vi "configuration UI.vi"() -> ()   [LabVIEW 2013, in "EIP Tags editor node.lvclass"]
uses:
  EIP Tags editor node.lvclass
  <vilib>/CEF_TreeControl/Node/NodeRef.ctl
  <vilib>/CEF_TreeControl/Node/NISE_CEF_Node.lvclass
  <vilib>/NI/AMC/Message Queue.ctl
  <vilib>/NI/AMC/Message.ctl
  <vilib>/NI/Tools/Keyed Array/KeyedArray.ctl
  <vilib>/CEF_TreeControl/Node/UserEventRef.ctl
  <vilib>/CEF_TreeControl/Controls/EventCluster.ctl
  <vilib>/NI/Tag Bus Data Framework/Configuration Editor/Classes/Engine Parent/Engine Parent Editor Node.lvclass
  <vilib>/NI/Tag Bus/tag/tag descriptor.lvclass
  <vilib>/NI/Tag Bus/tag/Data Type.ctl
  <vilib>/NI/Module Execution Interface/Engine Configuration/engine configuration.lvclass
  <vilib>/NI/TBM Modules/EIP Tags/configuration/EIP Tags Configuration.lvclass
  <vilib>/NI/Tag Bus/tag/tag descriptor.lvclass/tag descriptor.ctl
  EIP Tags editor node.lvclass/EIP Tags editor node.ctl
  <vilib>/NI/TBM Modules/EIP Tags/configuration/eip tag definition.ctl
  <vilib>/NI/TBM Modules/EIP Tags/configuration/eip tag types.ctl
  <vilib>/NI/Tag Bus Module Framework/root configuration/TBM configuration.lvclass/TBM configuration.ctl
  <vilib>/NI/Tag Bus/tag/write tag name.vi
  <vilib>/NI/Tag Bus/tag/write data type.vi
  <vilib>/NI/Tag Bus Data Framework/Configuration Editor/Classes/Module editor node/Read Module Configuration.vi
  <vilib>/NI/Tag Bus Module Framework/root configuration/create GUID.vi
  <vilib>/NI/Tag Bus Module Framework/module configuration/TBM module configuration.lvclass
  <vilib>/CEF_TreeControl/NISE_CEF_TreeControl.lvlib
  <vilib>/NI/Tag Bus Data Framework/Configuration Editor/Classes/Module editor node/module editor node.lvclass
  <vilib>/NI/Tag Bus Module Framework/root configuration/TBM configuration.lvclass
  <vilib>/NI/Tools/Keyed Array/Tools_KeyedArray.lvlib
  <vilib>/NI/AMC/AMC.lvlib
panel:
  in  "hidden_add":bool
  in  "Tab Control":enum32{"EIP Tags", "Channels"}(tab)
  in  "configure EIPT":bool
  in  "Remove EIPT":bool
  in  "Add EIPT":bool
  in  "EIP tags":i32(listbox)
  in  "Remove Button":bool
  in  "Add Button":bool
  in  "channel":i32(listbox)
  in  "settings":bool
  in  "user event":T1
  in  "main queue":T2
  in  "node ref":T3
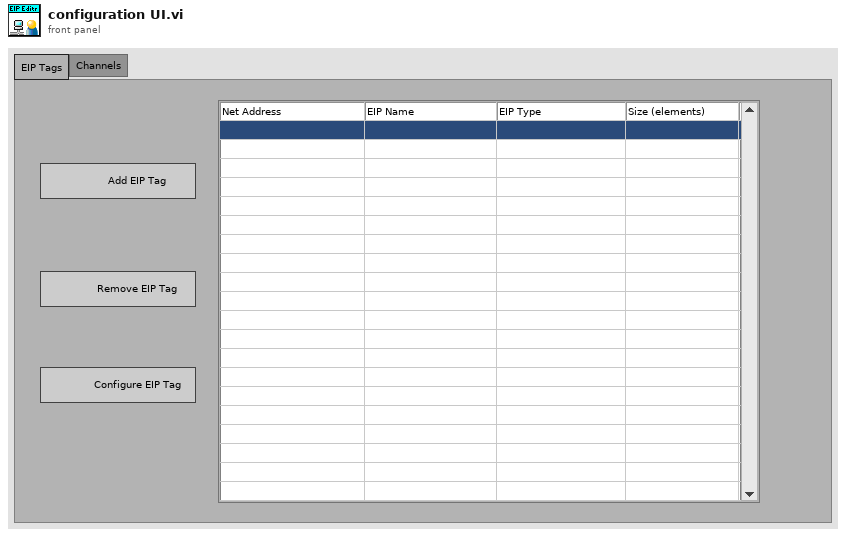
[diagram p1: front panel]
types:
  T1 = typedef "NISE_CEF_Node.lvclass/UserEventRef.ctl" = refnum<user-event>
  T2 = typedef "AMC.lvlib/Message Queue.ctl" = refnum<queue>
  T3 = typedef "NISE_CEF_Node.lvclass/NodeRef.ctl" = refnum<data-value>
  T4 = typedef "NISE_CEF_TreeControl.lvlib/EventCluster.ctl" = cluster{"command":string, "data":string}
  T5 = typedef "tag bus.lvlib/tag descriptor.lvclass/Data Type.ctl" = enum16{"Double", "Single", "I64", "I32", "I16", "I8", "U64", "U32", "U16", "U8", "Boolean", "String", "Array of Double", "Array of Single", "Array of I64", "Array of I32", "Array of I16", "Array of I8", "Array of U64", "Array of U32", "Array of U16", "Array of U8", "Array of Boolean", "Array of String"}
  T6 = typedef "EIP Tags Configuration.lvclass/eip tag definition.ctl" = cluster{"eip tag types":T7, "unique tag name":string, "Number of Elements":u32}
  T7 = typedef "EIP Tags Configuration.lvclass/eip tag types.ctl" = enum16{"SINT", "INT", "DINT", "REAL", "BOOL", "STRING"}
  T8 = typedef "EIP Tags editor node.lvclass/table line.ctl" = cluster{"eip channel":refnum<class "EIP Tags Channel.lvclass">, "tag name":string}
  T9 = typedef "LVPoint32TypeDef.ctl" = cluster{"Horizontal":i32, "Vertical":i32}
  T10 = typedef "LVRowAndColumnTypeDef.ctl" = cluster{"Row":i32, "Column":i32}
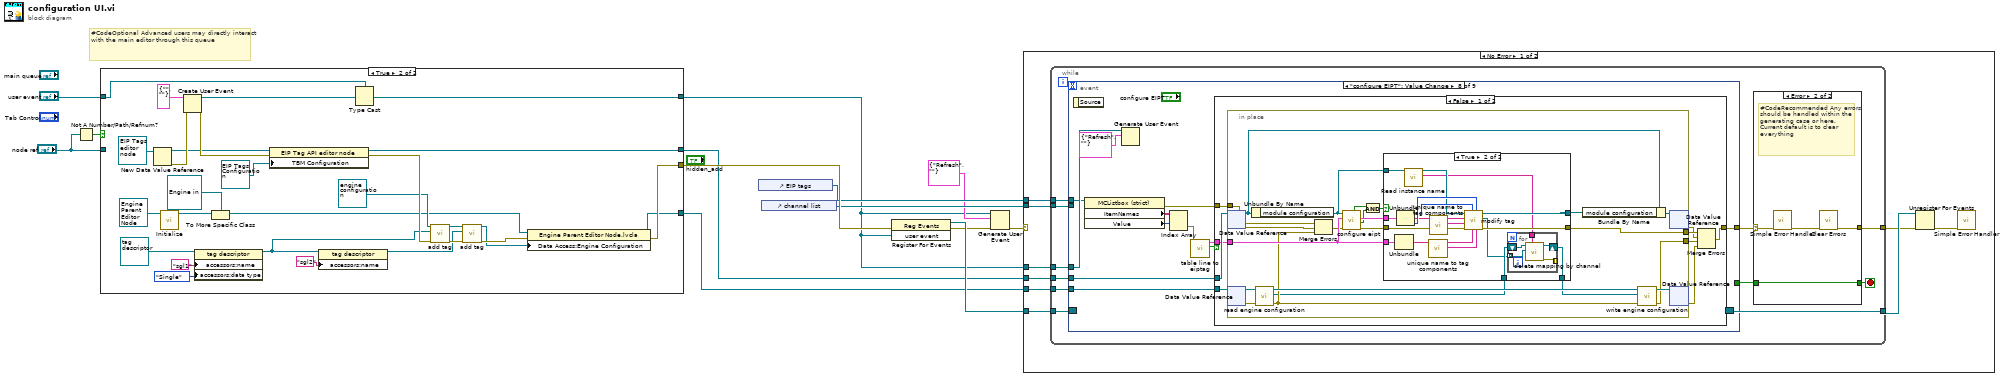
[diagram p0: block diagram]
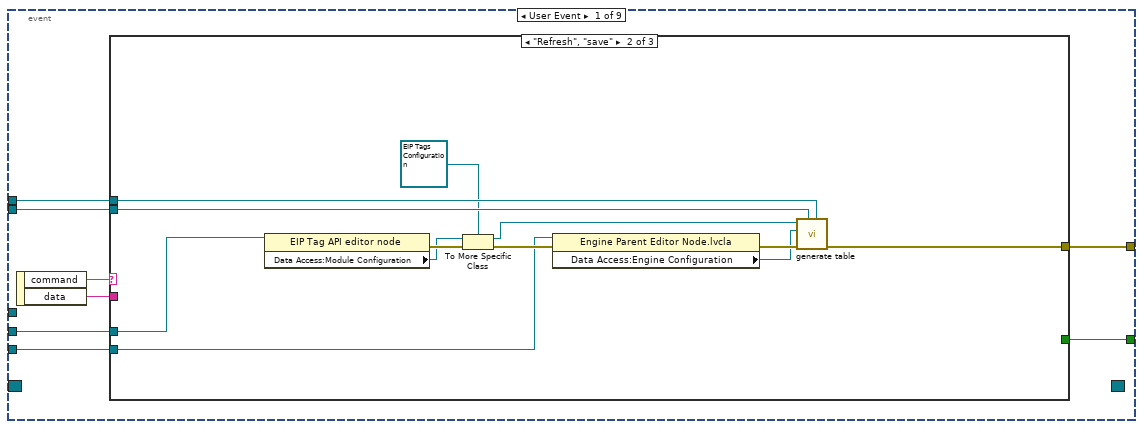
[diagram p3: hidden frame]
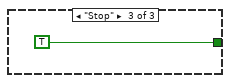
[diagram p5: hidden frame]
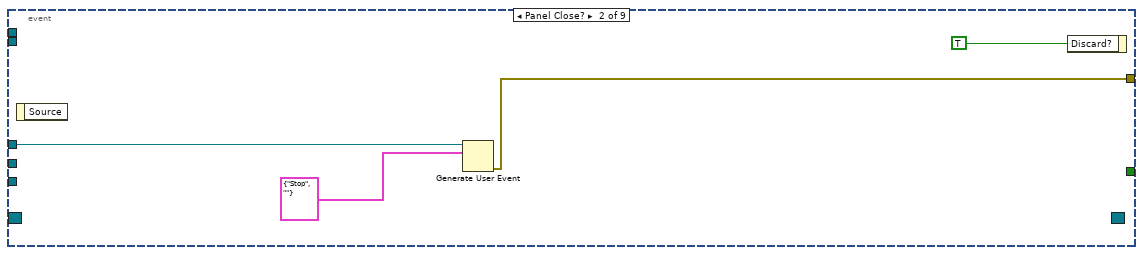
[diagram p6: hidden frame]
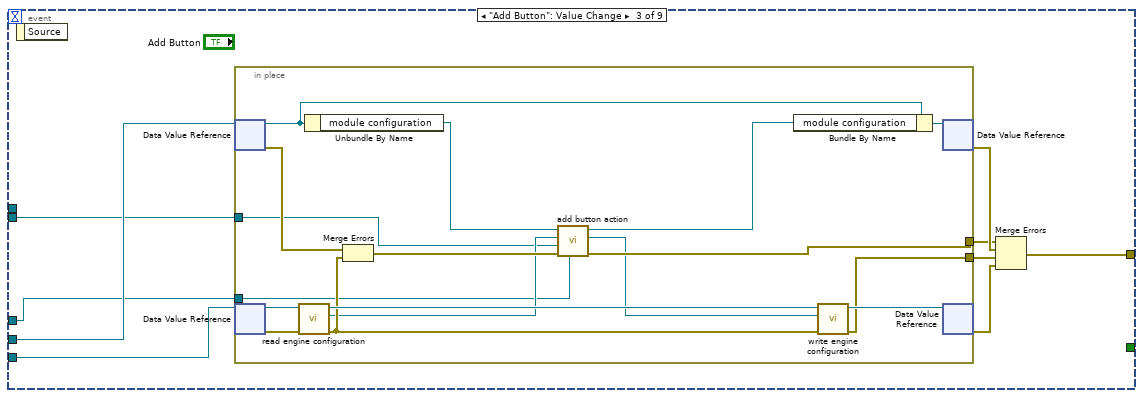
[diagram p7: hidden frame]
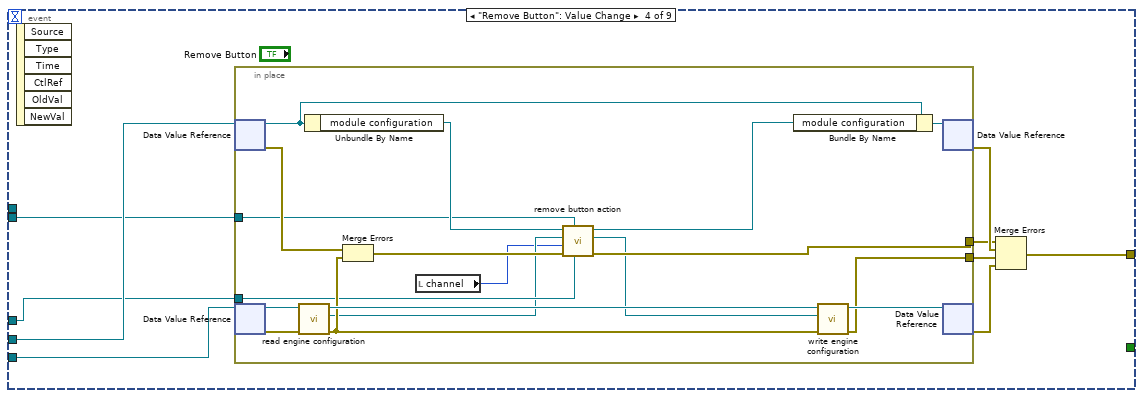
[diagram p8: hidden frame]
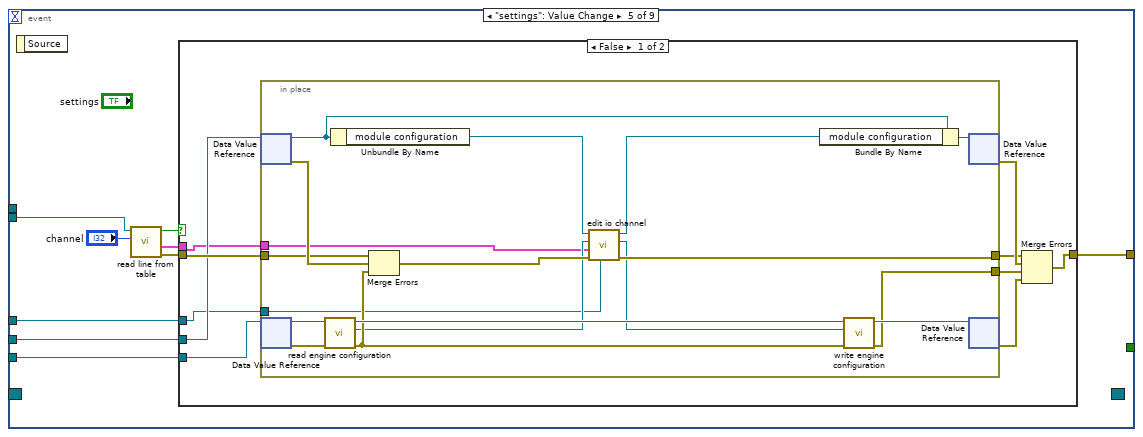
[diagram p9: hidden frame]
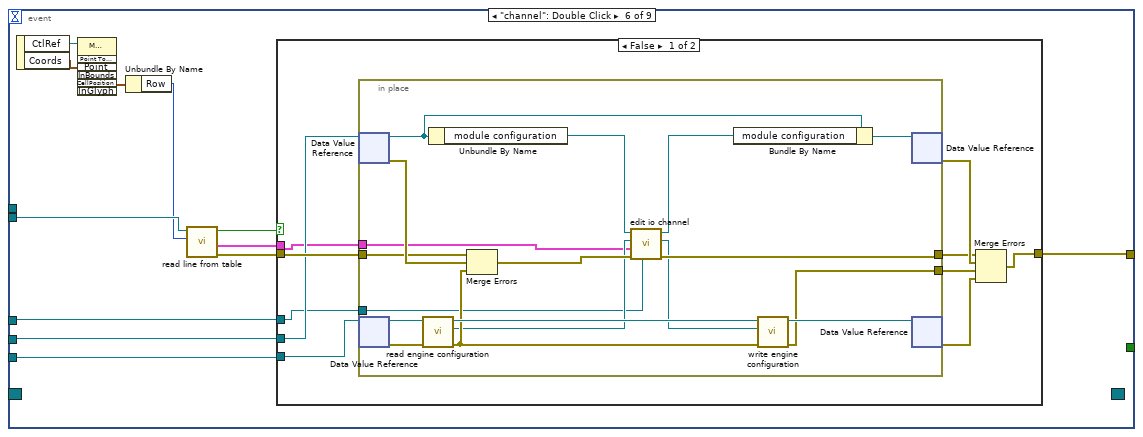
[diagram p11: hidden frame]
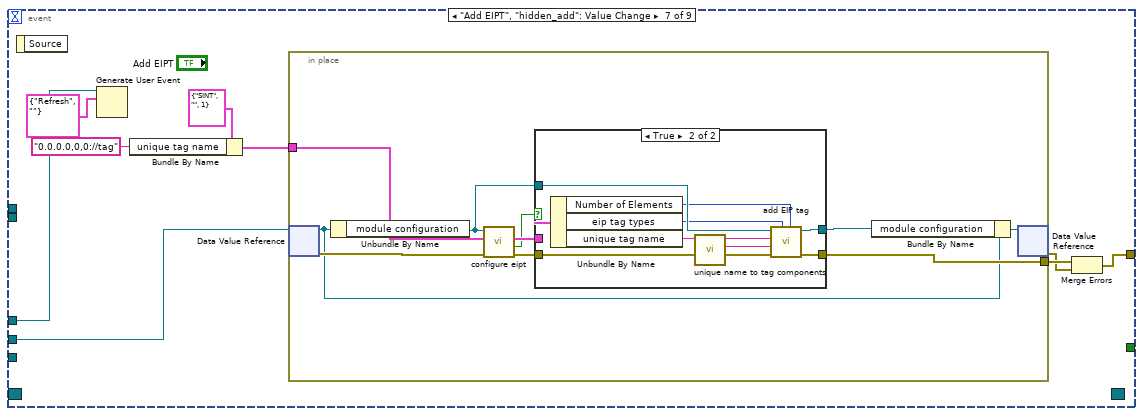
[diagram p13: hidden frame]
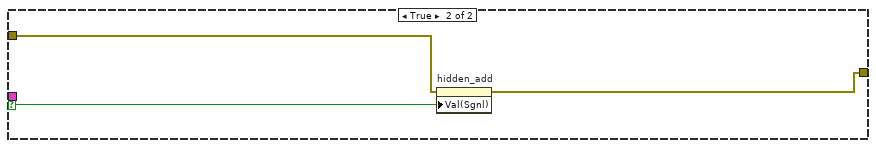
[diagram p16: hidden frame]
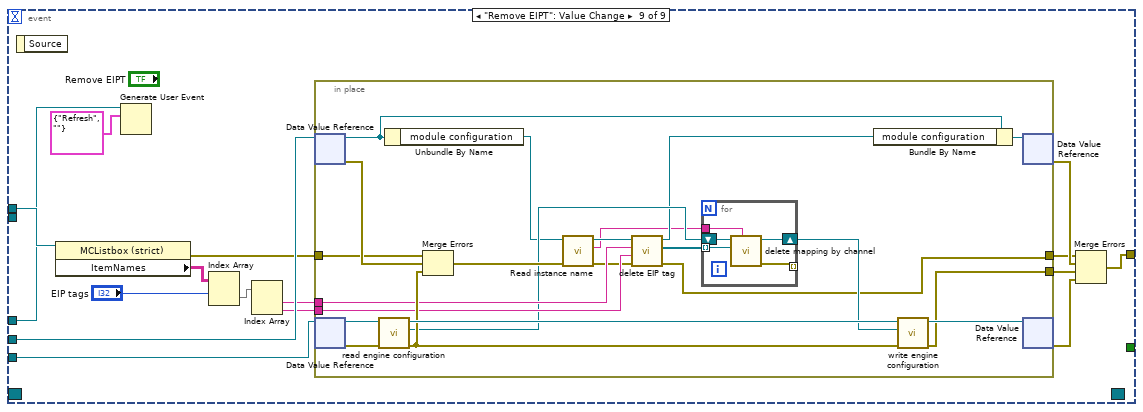
[diagram p17: hidden frame]
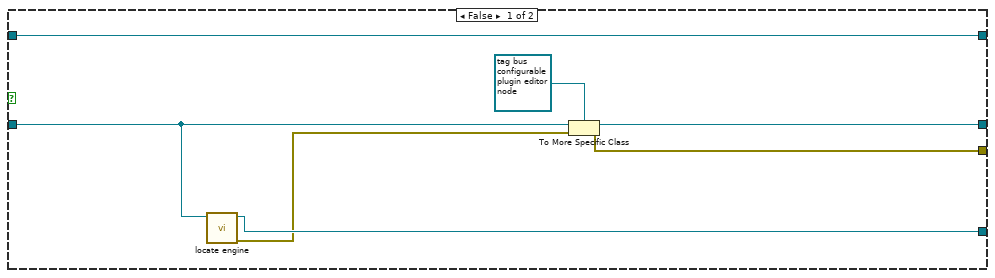
[diagram p19: hidden frame]
diagram:
  # "#CodeOptional Advanced users may directly interact with the main editor through this queue"
  n1 = Not A Number/Path/Refnum?(number/path/refnum="node ref") -> (NaN/Path/Refnum?=w12:bool)
  n2 = case shown="True" w12 {
    tunnel: "user event" -> [w20 w27]
    tunnel: [w20 w28] -> w3
    tunnel: "node ref" -> [w18 _]
    tunnel: [w17 w43] -> w8
    tunnel: [w16 w24] -> w10
    tunnel: [w15 w22] -> w7
    frame False {
      n3 = call <vilib>:"locate engine.vi"("component"=w18) -> ("error out"=w14:errorcluster, "engine"=w15:refnum<data-value>)  [unwired: 9 in]
      n4 = To More Specific Class(target class=refnum<data-value> refnum ("data value reference"), reference=w18, error in=w14) -> (specific class reference=w17:refnum<data-value>, error out=w16:errorcluster)
    }
    frame True {
      n5 = New Data Value Reference(data value=refnum<class "EIP Tags editor node.lvclass"> refnum ("tag bus configurable plugin editor node")) -> (data value reference=w42:refnum<data-value>, error out=w45:errorcluster)  [unwired: 1 in]
      n6 = call-dynamic "Initialize.vi"("Engine in"=refnum<class "Engine Parent Editor Node.lvclass"> refnum) -> ("data value reference"=w41:T3)  [unwired: 8 in, 2 out]
      n7 = Create User Event(user event datatype=T4 {"command"="", "data"=""} ("event data"), error in=w45) -> (user event=w47:refnum<user-event>, error out=w44:errorcluster)
      n8 = property class="tag descriptor"(reference=refnum<class "tag descriptor.lvclass"> refnum ("tag descriptor"), "accessors:name"="sgl1" ("name"), "accessors:data type"=Data_Type."Single" ("data type")) -> (reference out=w29:refnum<class "tag descriptor.lvclass">)  [unwired: 1 in, 1 out]
      n9 = To More Specific Class(target class=refnum<data-value> refnum ("data value reference"), reference=w41) -> (specific class reference=w23:refnum<data-value>)  [unwired: 1 in, 1 out]
      n10 = property class="EIP Tag API editor node"(reference=w42, error in=w44, "TBM Configuration"=refnum<class "EIP Tags Configuration.lvclass"> refnum ("tag bus configurable plugin module configuration")) -> (reference out=w43:refnum<data-value>, error out=w35:errorcluster)
      n11 = property class="tag descriptor"(reference=w29, "accessors:name"="sgl2" ("name")) -> (reference out=w30:refnum<class "tag descriptor.lvclass">)  [unwired: 1 in, 1 out]
      n12 = Type Cast(type=w27, x=w47) -> (*(type *) &x=w28:T1)
      n13 = call <vilib>:"add tag.vi"("error in"=w35, "tag descriptor"=w29, "engine configuration in"=refnum<class "engine configuration.lvclass"> refnum ("Engine Configuration")) -> ("error out"=w33:errorcluster, "engine configuration out"=w32:refnum<class "engine configuration.lvclass">)  [unwired: 7 in]
      n14 = call <vilib>:"add tag.vi"("error in"=w33, "tag descriptor"=w30, "engine configuration in"=w32) -> ("error out"=w31:errorcluster, "engine configuration out"=w21:refnum<class "engine configuration.lvclass">)  [unwired: 7 in]
      n15 = property class="Engine Parent Editor Node.lvcla"(reference=w23, error in=w31, "Data Access:Engine Configuration"=w21) -> (reference out=w22:refnum<data-value>, error out=w24:errorcluster)
    }
  }
  n16 = control-ref of="EIP tags"() -> (w5:refnum<vi>)
  n17 = control-ref of="channel list"() -> (w6:refnum<vi>)
  n18 = register-events(error in=w10, w3) -> (reference out=w13:refnum<event-registration>, error out=w2:errorcluster)  [unwired: 1 in]
  n19 = Generate User Event(user event=w3, event data cluster=T4 {"command"="Refresh", "data"=""} ("event data"), error in=w2) -> (error out=w1:errorcluster)  [unwired: 1 in, 1 out]
  n20 = case shown="No Error" w1 {
    tunnel: w13 -> [w57 _]
    tunnel: w8 -> [w54 _]
    tunnel: w7 -> [w53 _]
    tunnel: w6 -> [w51 _]
    tunnel: w5 -> [w50 _]
    tunnel: w3 -> [w49 _]
    frame No Error {
      n21 = while {
        tunnel: w57 -> [w68]
        tunnel: [w67] -> w56
        tunnel: w54 -> [w63]
        tunnel: w53 -> [w62]
        tunnel: w49 -> [w61]
        tunnel: w51 -> [w59]
        tunnel: w50 -> [w58]
        tunnel: [w64] -> w55
        stop <- w66 stop-if-true
        n22 = event shown="[7] \"configure EIPT\": Value Change" {
          selector: w68 -> [_ _ _ _ _ _ _ _ _]
          dyn-events: [_ _ _ _ _ _ _ _ _] -> w67
          timeout: _ -> [_ _ _ _ _ _ _ _ _]
          tunnel: [w82 _ _ _ _ _ _ _ _] -> w65
          tunnel: [w77 w96 w104 w130 w161 w194 w233 w271 w341] -> w60
          tunnel: w63 -> [w80 _ w102 w128 w153 w192 w234 w272 w339]
          tunnel: w62 -> [w79 _ w103 w129 w154 w191 _ w264 w340]
          tunnel: w61 -> [_ w98 w100 w126 w157 w193 w237 w273 w348]
          tunnel: w59 -> [w76 _ w101 w127 w155 w202 _ _ _]
          tunnel: w58 -> [w75 _ _ _ _ _ _ w270 w351]
          event User Event {
            n23 = event-data() -> ("command"=w81:string, "data"=w78:string)  [unwired: 1 in]
            n24 = case shown="\"Refresh\", \"save\"" w81 {
              tunnel: [_ _ TRUE] -> w82
              tunnel: w80 -> [_ w89 _]
              tunnel: w79 -> [_ w84 _]
              tunnel: w78 -> [_ _ _]
              tunnel: [_ w94 _] -> w77
              tunnel: w76 -> [_ w93 _]
              tunnel: w75 -> [_ w92 _]
              frame Default {
              }
              frame "Refresh", "save" {
                n25 = property class="EIP Tag API editor node"(reference=w89) -> (error out=w90:errorcluster, "Data Access:Module Configuration"=w87:refnum<class "TBM module configuration.lvclass">)  [unwired: 1 in, 1 out]
                n26 = To More Specific Class(target class=refnum<class "EIP Tags Configuration.lvclass"> refnum ("tag bus configurable plugin module configuration"), reference=w87, error in=w90) -> (specific class reference=w85:refnum<class "EIP Tags Configuration.lvclass">, error out=w88:errorcluster)
                n27 = property class="Engine Parent Editor Node.lvcla"(reference=w84, error in=w88) -> (error out=w91:errorcluster, "Data Access:Engine Configuration"=w83:refnum<class "engine configuration.lvclass">)  [unwired: 1 out]
                n28 = call "generate table.vi"("assemblies"=w92, "table"=w93, "error in"=w91, "engine configuration in"=w83, "EthernetIP configuration in"=w85) -> ("error out"=w94:errorcluster)  [unwired: 6 in]
              }
              frame "Stop" {
              }
            }
          }
          event Panel Close? {
            n29 = event-data() -> ()  [unwired: 1 in, 1 out]
            n30 = Generate User Event(user event=w98, event data cluster=T4 {"command"="Stop", "data"=""} ("event data")) -> (error out=w96:errorcluster)  [unwired: 2 in, 1 out]
            n31 = event-data("Discard?"=TRUE) -> ()  [unwired: 1 in, 1 out]
          }
          event "Add Button": Value Change {
            n32 = event-data() -> ()  [unwired: 1 in, 1 out]
            n33 = in-place {
              in-place-border: [w115] -> w105
              in-place-border: [w121] -> w108
              in-place-border: w101 -> [w110]
              in-place-border: w100 -> [w109]
              n34 = in-place-dvr #1(w102) -> (w125:refnum<class "EIP Tags editor node.lvclass">, w123:errorcluster)
              n35 = in-place-dvr #2(w103) -> (w120:refnum<class "Engine Parent Editor Node.lvclass">, w119:errorcluster)
              n36 = call <vilib>:"read engine configuration.vi"("error in"=w119, "Engine Parent Editor Node in"=w120) -> ("error out"=w117:errorcluster, "engine configuration"=w112:refnum<class "engine configuration.lvclass">, "Engine Parent Editor Node out"=w118:refnum<class "Engine Parent Editor Node.lvclass">)  [unwired: 7 in]
              n37 = Unbundle By Name(w125) -> ("module configuration"=w113:refnum<class "EIP Tags Configuration.lvclass">)
              n38 = Merge Errors(w123, w117) -> (w116:errorcluster)
              n39 = call "add button action.vi"("user event"=w109, "error in"=w116, "channel list"=w110, "Engine Configuration"=w112, "EIP Tags Configuration in"=w113) -> ("error out"=w115:errorcluster, "Engine Configuration out"=w111:refnum<class "engine configuration.lvclass">, "module configuration out"=w114:refnum<class "EIP Tags Configuration.lvclass">)  [unwired: 4 in]
              n40 = Bundle By Name(cluster=w125, "module configuration"=w114) -> (w124:refnum<class "EIP Tags editor node.lvclass">)
              n41 = call <vilib>:"write engine configuration.vi"("error in"=w117, "engine configuration"=w111, "Engine Parent Editor Node in"=w118) -> ("error out"=w121:errorcluster, "Engine Parent Editor Node out"=w122:refnum<class "Engine Parent Editor Node.lvclass">)  [unwired: 7 in]
              n42 = in-place-dvr #1(w124) -> (w107:errorcluster)  [unwired: 1 out]
              n43 = in-place-dvr #2(w122) -> (w106:errorcluster)  [unwired: 1 out]
            }
            n44 = Merge Errors(w105, w107, w108, w106) -> (w104:errorcluster)
          }
          event "Remove Button": Value Change {
            n45 = event-data() -> ()  [unwired: 1 in, 6 out]
            n46 = in-place {
              in-place-border: [w142] -> w131
              in-place-border: [w148] -> w134
              in-place-border: w127 -> [w138]
              in-place-border: w126 -> [w141]
              n47 = in-place-dvr #3(w128) -> (w152:refnum<class "EIP Tags editor node.lvclass">, w150:errorcluster)
              n48 = in-place-dvr #4(w129) -> (w147:refnum<class "Engine Parent Editor Node.lvclass">, w146:errorcluster)
              n49 = call <vilib>:"read engine configuration.vi"("error in"=w146, "Engine Parent Editor Node in"=w147) -> ("error out"=w144:errorcluster, "engine configuration"=w137:refnum<class "engine configuration.lvclass">, "Engine Parent Editor Node out"=w145:refnum<class "Engine Parent Editor Node.lvclass">)  [unwired: 7 in]
              n50 = Unbundle By Name(w152) -> ("module configuration"=w139:refnum<class "EIP Tags Configuration.lvclass">)
              n51 = Merge Errors(w150, w144) -> (w143:errorcluster)
              n52 = local read "channel"() -> (w135:i32)
              n53 = call "remove button action.vi"("user event"=w141, "channel list"=w138, "error in"=w143, "channel"=w135, "Engine Configuration in"=w137, "EIP Tags Configuration in"=w139) -> ("error out"=w142:errorcluster, "Engine Configuration out"=w136:refnum<class "engine configuration.lvclass">, "EIP Tags Configuration out"=w140:refnum<class "EIP Tags Configuration.lvclass">)  [unwired: 3 in]
              n54 = Bundle By Name(cluster=w152, "module configuration"=w140) -> (w151:refnum<class "EIP Tags editor node.lvclass">)
              n55 = call <vilib>:"write engine configuration.vi"("error in"=w144, "engine configuration"=w136, "Engine Parent Editor Node in"=w145) -> ("error out"=w148:errorcluster, "Engine Parent Editor Node out"=w149:refnum<class "Engine Parent Editor Node.lvclass">)  [unwired: 7 in]
              n56 = in-place-dvr #3(w151) -> (w133:errorcluster)  [unwired: 1 out]
              n57 = in-place-dvr #4(w149) -> (w132:errorcluster)  [unwired: 1 out]
            }
            n58 = Merge Errors(w131, w133, w134, w132) -> (w130:errorcluster)
          }
          event "settings": Value Change {
            n59 = event-data() -> ()  [unwired: 1 in, 1 out]
            n60 = call "read line from table.vi"("line number"="channel", "channels table"=w155) -> ("error out"=w160:errorcluster, "line"=w159:T8, "empty channel?"=w156:bool)  [unwired: 6 in, 1 out]
            n61 = case shown="False" w156 {
              tunnel: [w167 w190] -> w161
              tunnel: w160 -> [w166 w190]
              tunnel: w159 -> [w163 _]
              tunnel: w157 -> [w162 _]
              tunnel: w154 -> [w165 _]
              tunnel: w153 -> [w164 _]
              frame False {
                n62 = in-place {
                  in-place-border: [w178] -> w168
                  in-place-border: [w185] -> w171
                  in-place-border: w166 -> [w180]
                  in-place-border: w163 -> [w173]
                  in-place-border: w162 -> [w172]
                  n63 = in-place-dvr #5(w164) -> (w189:refnum<class "EIP Tags editor node.lvclass">, w187:errorcluster)
                  n64 = in-place-dvr #6(w165) -> (w184:refnum<class "Engine Parent Editor Node.lvclass">, w183:errorcluster)
                  n65 = call <vilib>:"read engine configuration.vi"("error in"=w183, "Engine Parent Editor Node in"=w184) -> ("error out"=w181:errorcluster, "engine configuration"=w174:refnum<class "engine configuration.lvclass">, "Engine Parent Editor Node out"=w182:refnum<class "Engine Parent Editor Node.lvclass">)  [unwired: 7 in]
                  n66 = Unbundle By Name(w189) -> ("module configuration"=w177:refnum<class "EIP Tags Configuration.lvclass">)
                  n67 = Merge Errors(w180, w187, w181) -> (w179:errorcluster)
                  n68 = call "edit io channel.vi"("user event"=w172, "error in"=w179, "line"=w173, "engine configuration in"=w174, "EthernetIP configuration in"=w177) -> ("error out"=w178:errorcluster, "engine configuration out"=w175:refnum<class "engine configuration.lvclass">, "EthernetIP configuration out"=w176:refnum<class "EIP Tags Configuration.lvclass">)  [unwired: 4 in]
                  n69 = Bundle By Name(cluster=w189, "module configuration"=w176) -> (w188:refnum<class "EIP Tags editor node.lvclass">)
                  n70 = call <vilib>:"write engine configuration.vi"("error in"=w181, "engine configuration"=w175, "Engine Parent Editor Node in"=w182) -> ("error out"=w185:errorcluster, "Engine Parent Editor Node out"=w186:refnum<class "Engine Parent Editor Node.lvclass">)  [unwired: 7 in]
                  n71 = in-place-dvr #5(w188) -> (w170:errorcluster)  [unwired: 1 out]
                  n72 = in-place-dvr #6(w186) -> (w169:errorcluster)  [unwired: 1 out]
                }
                n73 = Merge Errors(w168, w170, w171, w169) -> (w167:errorcluster)
              }
              frame True {
              }
            }
          }
          event "channel": Double Click {
            n74 = event-data() -> ("CtlRef"=w201:refnum<vi>, "Coords"=w200:T9)  [unwired: 1 in]
            n75 = invoke class="MCListbox (strict)" method="Point To Row Column"(reference=w201, "Point"=w200) -> ("CellPosition"=w199:T10)  [unwired: 5 in, 6 out]
            n76 = Unbundle By Name(w199) -> ("Row"=w198:i32)
            n77 = call "read line from table.vi"("line number"=w198, "channels table"=w202) -> ("error out"=w197:errorcluster, "line"=w196:T8, "empty channel?"=w195:bool)  [unwired: 6 in, 1 out]
            n78 = case shown="False" w195 {
              tunnel: [w208 w231] -> w194
              tunnel: w197 -> [w207 w231]
              tunnel: w196 -> [w204 _]
              tunnel: w193 -> [w203 _]
              tunnel: w191 -> [w206 _]
              tunnel: w192 -> [w205 _]
              frame False {
                n79 = in-place {
                  in-place-border: [w219] -> w209
                  in-place-border: [w226] -> w212
                  in-place-border: w207 -> [w221]
                  in-place-border: w204 -> [w214]
                  in-place-border: w203 -> [w213]
                  n80 = in-place-dvr #7(w205) -> (w230:refnum<class "EIP Tags editor node.lvclass">, w228:errorcluster)
                  n81 = in-place-dvr #8(w206) -> (w225:refnum<class "Engine Parent Editor Node.lvclass">, w224:errorcluster)
                  n82 = call <vilib>:"read engine configuration.vi"("error in"=w224, "Engine Parent Editor Node in"=w225) -> ("error out"=w222:errorcluster, "engine configuration"=w215:refnum<class "engine configuration.lvclass">, "Engine Parent Editor Node out"=w223:refnum<class "Engine Parent Editor Node.lvclass">)  [unwired: 7 in]
                  n83 = Unbundle By Name(w230) -> ("module configuration"=w218:refnum<class "EIP Tags Configuration.lvclass">)
                  n84 = Merge Errors(w221, w228, w222) -> (w220:errorcluster)
                  n85 = call "edit io channel.vi"("user event"=w213, "error in"=w220, "line"=w214, "engine configuration in"=w215, "EthernetIP configuration in"=w218) -> ("error out"=w219:errorcluster, "engine configuration out"=w216:refnum<class "engine configuration.lvclass">, "EthernetIP configuration out"=w217:refnum<class "EIP Tags Configuration.lvclass">)  [unwired: 4 in]
                  n86 = Bundle By Name(cluster=w230, "module configuration"=w217) -> (w229:refnum<class "EIP Tags editor node.lvclass">)
                  n87 = call <vilib>:"write engine configuration.vi"("error in"=w222, "engine configuration"=w216, "Engine Parent Editor Node in"=w223) -> ("error out"=w226:errorcluster, "Engine Parent Editor Node out"=w227:refnum<class "Engine Parent Editor Node.lvclass">)  [unwired: 7 in]
                  n88 = in-place-dvr #7(w229) -> (w211:errorcluster)  [unwired: 1 out]
                  n89 = in-place-dvr #8(w227) -> (w210:errorcluster)  [unwired: 1 out]
                }
                n90 = Merge Errors(w209, w211, w212, w210) -> (w208:errorcluster)
              }
              frame True {
              }
            }
          }
          event "Add EIPT", "hidden_add": Value Change {
            n91 = event-data() -> ()  [unwired: 1 in, 1 out]
            n92 = Generate User Event(user event=w237, event data cluster=T4 {"command"="Refresh", "data"=""} ("event data")) -> ()  [unwired: 2 in, 2 out]
            n93 = Bundle By Name(cluster=T6 {"eip tag types"=enum."SINT", "unique tag name"="", "Number of Elements"=1} ("tag spec"), "unique tag name"="0.0.0.0,0,0://tag") -> (w239:T6)
            n94 = in-place {
              in-place-border: [w249] -> w240
              in-place-border: w239 -> [w246]
              n95 = in-place-dvr #9(w234) -> (w243:refnum<class "EIP Tags editor node.lvclass">, w245:errorcluster)
              n96 = Unbundle By Name(w243) -> ("module configuration"=w241:refnum<class "EIP Tags Configuration.lvclass">)
              n97 = call "configure eipt.vi"("error in"=w245, "tag definition in"=w246, "EthernetIP configuration"=w241) -> ("error out"=w250:errorcluster, "success"=w247:bool, "tag definition out"=w248:T6)  [unwired: 5 in, 1 out]
              n98 = case shown="True" w247 {
                tunnel: w250 -> [w251 w262]
                tunnel: [w251 w261] -> w249
                tunnel: [w252 w260] -> w242
                tunnel: w241 -> [w252 w259]
                tunnel: w248 -> [_ w258]
                frame False {
                }
                frame True {
                  n99 = Unbundle By Name(w258) -> ("Number of Elements"=w256:u32, "eip tag types"=w257:T7, "unique tag name"=w255:string)
                  n100 = call <vilib>:"unique name to tag components.vi"("unique name"=w255) -> ("Tag Name"=w253:string, "Network Path"=w254:string)  [unwired: 9 in]
                  n101 = call <vilib>:"add EIP tag.vi"("Number of Elements"=w256, "eip tag types"=w257, "error in"=w262, "Tag Name"=w253, "Network Path"=w254, "EIP Tags configuration in"=w259) -> ("error out"=w261:errorcluster, "EIP Tags configuration out"=w260:refnum<class "EIP Tags Configuration.lvclass">)  [unwired: 4 in]
                }
              }
              n102 = Bundle By Name(cluster=w243, "module configuration"=w242) -> (w244:refnum<class "EIP Tags editor node.lvclass">)
              n103 = in-place-dvr #9(w244) -> (w232:errorcluster)  [unwired: 1 out]
            }
            n104 = Merge Errors(w240, w232) -> (w233:errorcluster)
          }
          event "configure EIPT": Value Change {
            n105 = event-data() -> ()  [unwired: 1 in, 1 out]
            n106 = property class="MCListbox (strict)"(reference=w270) -> (error out=w263:errorcluster, "ItemNames"=w269:string[][], "Value"=w268:i32)  [unwired: 1 in, 1 out]
            n107 = Generate User Event(user event=w273, event data cluster=T4 {"command"="Refresh", "data"=""} ("event data")) -> ()  [unwired: 2 in, 2 out]
            n108 = Index Array(array=w269, index (row)=w268) -> (element=w267:string[])  [unwired: 1 in]
            n109 = call "table line to eiptag.vi"("line strings"=w267) -> ("invalid?"=w266:bool, "tag"=w265:T6)  [unwired: 9 in]
            n110 = case shown="False" w266 {
              selector: w266 -> [_ w335]
              tunnel: w272 -> [w282 _]
              tunnel: [w281 w334] -> w271
              tunnel: w265 -> [w279 _]
              tunnel: w264 -> [w278 _]
              tunnel: w263 -> [w275 w333]
              frame False {
                n111 = in-place {
                  in-place-border: [w304] -> w283
                  in-place-border: w279 -> [w294]
                  in-place-border: [w287] -> w276
                  in-place-border: w275 -> [w284]
                  n112 = in-place-dvr #10(w282) -> (w300:refnum<class "EIP Tags editor node.lvclass">, w302:errorcluster)
                  n113 = in-place-dvr #11(w278) -> (w293:refnum<class "Engine Parent Editor Node.lvclass">, w292:errorcluster)
                  n114 = Unbundle By Name(w300) -> ("module configuration"=w298:refnum<class "EIP Tags Configuration.lvclass">)
                  n115 = call <vilib>:"read engine configuration.vi"("error in"=w292, "Engine Parent Editor Node in"=w293) -> ("error out"=w288:errorcluster, "engine configuration"=w286:refnum<class "engine configuration.lvclass">, "Engine Parent Editor Node out"=w289:refnum<class "Engine Parent Editor Node.lvclass">)  [unwired: 7 in]
                  n116 = Merge Errors(w284, w302, w288) -> (w291:errorcluster)
                  n117 = call "configure eipt.vi"("error in"=w291, "tag definition in"=w294, "EthernetIP configuration"=w298) -> ("error out"=w305:errorcluster, "success"=w295:bool, "tag definition out"=w303:T6, "changed"=w296:bool)  [unwired: 5 in]
                  n118 = And(x=w296, y=w295) -> (x .and. y?=w297:bool)
                  n119 = case shown="True" w297 {
                    tunnel: w305 -> [w307 w327]
                    tunnel: [w307 w326] -> w304
                    tunnel: [w308 w325] -> w299
                    tunnel: w298 -> [w308 w312]
                    tunnel: w303 -> [_ w323]
                    tunnel: w294 -> [_ w324]
                    tunnel: w286 -> [w306 w314]
                    tunnel: [w306 w313] -> w285
                    frame False {
                    }
                    frame True {
                      n120 = Unbundle(w324) -> ("unique tag name"=w317:string)  [unwired: 2 out]
                      n121 = Unbundle(w323) -> ("eip tag types"=w321:T7, "unique tag name"=w320:string, "Number of Elements"=w322:u32)
                      n122 = call <vilib>:"Read instance name.vi"("configuration in"=w312) -> ("instance id"=w310:string, "configuration out"=w311:refnum<class "EIP Tags Configuration.lvclass">)  [unwired: 8 in, 1 out]
                      n123 = call <vilib>:"unique name to tag components.vi"("unique name"=w317) -> ("Tag Name"=w315:string, "Network Path"=w316:string)  [unwired: 9 in]
                      n124 = call <vilib>:"unique name to tag components.vi"("unique name"=w320) -> ("Tag Name"=w318:string, "Network Path"=w319:string)  [unwired: 9 in]
                      n125 = call <vilib>:"modify tag.vi"("original tag name"=w315, "Number of Elements"=w322, "original network path"=w316, "eip tag types"=w321, "error in"=w327, "Tag Name"=w318, "Network Path"=w319, "EIP Tags configuration in"=w311) -> ("error out"=w326:errorcluster, "removed channels"=w309:refnum<class "EIP Tags Channel.lvclass">[], "EIP Tags configuration out"=w325:refnum<class "EIP Tags Configuration.lvclass">)  [unwired: 1 in]
                      n126 = for {
                        shift-right: [w332] -> w313
                        shift-left: w314 -> [w331]
                        tunnel: [w330] -> _ mode=indexing
                        tunnel: w310 -> [w329]
                        tunnel: w309 -> [w328] mode=indexing
                        n127 = call <vilib>:"delete mapping by channel.vi"("owner ID"=w329, "channel"=w328, "engine configuration in"=w331) -> ("error out"=w330:errorcluster, "engine configuration out"=w332:refnum<class "engine configuration.lvclass">)  [unwired: 7 in]
                      }
                    }
                  }
                  n128 = Bundle By Name(cluster=w300, "module configuration"=w299) -> (w301:refnum<class "EIP Tags editor node.lvclass">)
                  n129 = call <vilib>:"write engine configuration.vi"("error in"=w288, "engine configuration"=w285, "Engine Parent Editor Node in"=w289) -> ("error out"=w287:errorcluster, "Engine Parent Editor Node out"=w290:refnum<class "Engine Parent Editor Node.lvclass">)  [unwired: 7 in]
                  n130 = in-place-dvr #10(w301) -> (w280:errorcluster)  [unwired: 1 out]
                  n131 = in-place-dvr #11(w290) -> (w277:errorcluster)  [unwired: 1 out]
                }
                n132 = Merge Errors(w283, w280, w276, w277) -> (w281:errorcluster)
              }
              frame True {
                n133 = property on="hidden_add" class="Bool (strict)"(error in=w333, "Val(Sgnl)"=w335) -> (error out=w334:errorcluster)  [unwired: 1 in, 1 out]
              }
            }
          }
          event "Remove EIPT": Value Change {
            n134 = event-data() -> ()  [unwired: 1 in, 1 out]
            n135 = property class="MCListbox (strict)"(reference=w351) -> (error out=w338:errorcluster, "ItemNames"=w350:string[][])  [unwired: 1 in, 1 out]
            n136 = Generate User Event(user event=w348, event data cluster=T4 {"command"="Refresh", "data"=""} ("event data")) -> ()  [unwired: 2 in, 2 out]
            n137 = Index Array(array=w350, index (row)="EIP tags") -> (element=w346:string[])  [unwired: 1 in]
            n138 = Index Array(array=w346) -> (element #1=w337:string, element #2=w336:string)  [unwired: 2 in]
            n139 = in-place {
              in-place-border: [w352] -> w342
              in-place-border: [w369] -> w345
              in-place-border: w338 -> [w364]
              in-place-border: w337 -> [w362]
              in-place-border: w336 -> [w361]
              n140 = in-place-dvr #12(w339) -> (w373:refnum<class "EIP Tags editor node.lvclass">, w371:errorcluster)
              n141 = in-place-dvr #13(w340) -> (w368:refnum<class "Engine Parent Editor Node.lvclass">, w367:errorcluster)
              n142 = call <vilib>:"read engine configuration.vi"("error in"=w367, "Engine Parent Editor Node in"=w368) -> ("error out"=w365:errorcluster, "engine configuration"=w360:refnum<class "engine configuration.lvclass">, "Engine Parent Editor Node out"=w366:refnum<class "Engine Parent Editor Node.lvclass">)  [unwired: 7 in]
              n143 = Unbundle By Name(w373) -> ("module configuration"=w357:refnum<class "EIP Tags Configuration.lvclass">)
              n144 = Merge Errors(w364, w371, w365) -> (w363:errorcluster)
              n145 = call <vilib>:"Read instance name.vi"("error in"=w363, "configuration in"=w357) -> ("error out"=w355:errorcluster, "instance id"=w353:string, "configuration out"=w354:refnum<class "EIP Tags Configuration.lvclass">)  [unwired: 7 in]
              n146 = call <vilib>:"delete EIP tag.vi"("error in"=w355, "Tag Name"=w361, "Network Path"=w362, "EIP Tags configuration in"=w354) -> ("error out"=w352:errorcluster, "removed channels"=w356:refnum<class "EIP Tags Channel.lvclass">[], "EIP Tags configuration out"=w358:refnum<class "EIP Tags Configuration.lvclass">)  [unwired: 5 in]
              n147 = for {
                shift-right: [w378] -> w359
                shift-left: w360 -> [w377]
                tunnel: w356 -> [w376] mode=indexing
                tunnel: [w375] -> _ mode=indexing
                tunnel: w353 -> [w374]
                n148 = call <vilib>:"delete mapping by channel.vi"("owner ID"=w374, "channel"=w376, "engine configuration in"=w377) -> ("error out"=w375:errorcluster, "engine configuration out"=w378:refnum<class "engine configuration.lvclass">)  [unwired: 7 in]
              }
              n149 = Bundle By Name(cluster=w373, "module configuration"=w358) -> (w372:refnum<class "EIP Tags editor node.lvclass">)
              n150 = call <vilib>:"write engine configuration.vi"("error in"=w365, "engine configuration"=w359, "Engine Parent Editor Node in"=w366) -> ("error out"=w369:errorcluster, "Engine Parent Editor Node out"=w370:refnum<class "Engine Parent Editor Node.lvclass">)  [unwired: 7 in]
              n151 = in-place-dvr #12(w372) -> (w344:errorcluster)  [unwired: 1 out]
              n152 = in-place-dvr #13(w370) -> (w343:errorcluster)  [unwired: 1 out]
            }
            n153 = Merge Errors(w342, w344, w345, w343) -> (w341:errorcluster)
          }
        }
        n154 = case shown="Error" w60 {
          selector: w60 -> [w69 w73]
          tunnel: [w70 w74] -> w66
          tunnel: w65 -> [w70 w74]
          tunnel: [w69 w71] -> w64
          frame No Error {
          }
          frame Error {
            # "#CodeRecommended Any errors should be handled within the generating case or here. Current default is to clear everything"
            n155 = call <vilib>:"Simple Error Handler.vi"("error in (no error)"=w73) -> ("error out"=w72:errorcluster)  [unwired: 4 in, 4 out]
            n156 = call <vilib>:"Clear Errors.vi"("error in (no error)"=w72) -> ("error out"=w71:errorcluster)  [unwired: 6 in]
          }
        }
      }
      n157 = Unregister For Events(event registration refnum=w56, error in=w55) -> (error out=w52:errorcluster)
      n158 = call <vilib>:"Simple Error Handler.vi"("error in (no error)"=w52) -> ()  [unwired: 4 in, 5 out]
    }
    frame Error {
    }
  }
